vi "setROI.vi"(8 "error in (no error)":errorcluster, 10 "Coordinates":i32[](array[numeric]), 11 "ImageStreamViewer in":refnum<class "ImageStreamViewer.lvclass">) -> (0 "error out":errorcluster, 3 "ImageStreamViewer out":refnum<class "ImageStreamViewer.lvclass">)   [LabVIEW 2011, in "Views.lvlib" / "Camera.lvlib" / "ImageStreamViewer.lvclass"]
uses:
  ImageStreamViewer.lvclass
  ImageStreamViewer.lvclass/ImageStreamViewer.ctl
  Tools/Imaging.lvlib
panel:
  # "From the rectangle coordinates, redraw the ROI \nbox, and update the ROI file."
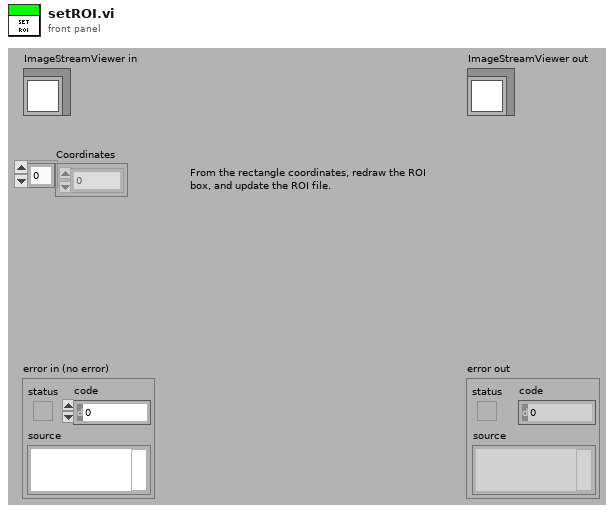
[diagram p1: front panel]
types:
  T1 = cluster{"Left":i32, "Top":i32, "Right":i32, "Bottom":i32}
  T2 = typedef "IMAQ Image.ctl" = refnum<image>
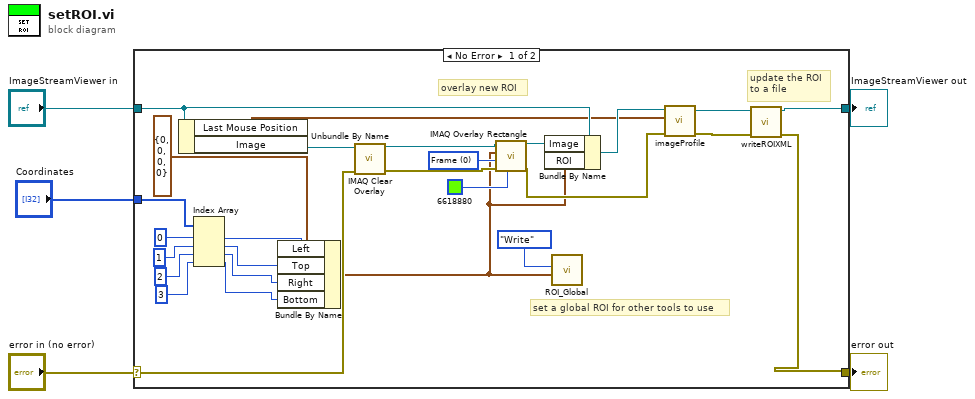
[diagram p0: block diagram]
diagram:
  n1 = case shown="No Error" "error in (no error)" {
    selector: "error in (no error)" -> [w16 w34]
    tunnel: [w9 w34] -> w4
    tunnel: [w8 w33] -> w2
    tunnel: "ImageStreamViewer in" -> [w24 w33]
    tunnel: "Coordinates" -> [w32 _]
    frame No Error {
      w27 = u32 0 items=["Frame", "Fill", "Highlight"] ("Drawing Mode (Frame)")
      # "overlay new ROI"
      # "set a global ROI for other tools to use"
      # "update the ROI\nto a file"
      n2 = Unbundle By Name(w24) -> ("Last Mouse Position"=w12:cluster{"X":i32, "Y":i32}, "Image"=w17:T2)
      n3 = Index Array(array=w32, index #1=0, index #2=1, index #3=2, index #4=3) -> (element #1=w23:i32, element #2=w22:i32, element #3=w21:i32, element #4=w20:i32)
      n4 = Bundle By Name(cluster=T1 {"Left"=0, "Top"=0, "Right"=0, "Bottom"=0} ("Rectangle"), "Left"=w23, "Top"=w22, "Right"=w21, "Bottom"=w20) -> (w6:T1)
      n5 = call "IMAQ Clear Overlay"("error in (no error)"=w16, "Image"=w17) -> ("error out"=w15:errorcluster, "Image Out"=w18:T2)  [unwired: 8 in]
      n6 = call "IMAQ Overlay Rectangle"("Color"=u32 6618880, "error in (no error)"=w15, "Drawing Mode (Frame)"=w27, "Rectangle"=w6, "Image"=w18) -> ("error out"=w13:errorcluster, "Image Out"=w25:T2)  [unwired: 5 in]
      n7 = Bundle By Name(cluster=w24, "Image"=w25, "ROI"=w6) -> (w14:refnum<class "ImageStreamViewer.lvclass">)
      n8 = call "ROI_Global.vi"("ROI"=w6, "Action"=enum16{"Write", "Read"}."Write") -> ()  [unwired: 9 in, 1 out]
      n9 = call "imageProfile.vi"("error in (no error)"=w13, "Point"=w12, "ImageStreamViewer in"=w14) -> ("error out"=w10:errorcluster, "ImageStreamViewer out"=w11:refnum<class "ImageStreamViewer.lvclass">)  [unwired: 7 in]
      n10 = call "writeROIXML.vi"("error in (no error)"=w10, "ImageStreamViewer in"=w11) -> ("error out"=w9:errorcluster, "ImageStreamViewer out"=w8:refnum<class "ImageStreamViewer.lvclass">)  [unwired: 8 in]
    }
    frame Error {
    }
  }
  "error out" <- w4
  "ImageStreamViewer out" <- w2
